vi "DI Remains.vi"(11 "DI":T1(array[cluster])) -> (2 "Same DI":T1(array[cluster]), 3 "Remains":T1(array[cluster]), 4 "DI Index":i32[](array[numeric]), 5 "DI value":bool[](array[boolean]))   [LabVIEW 2022 SP3]
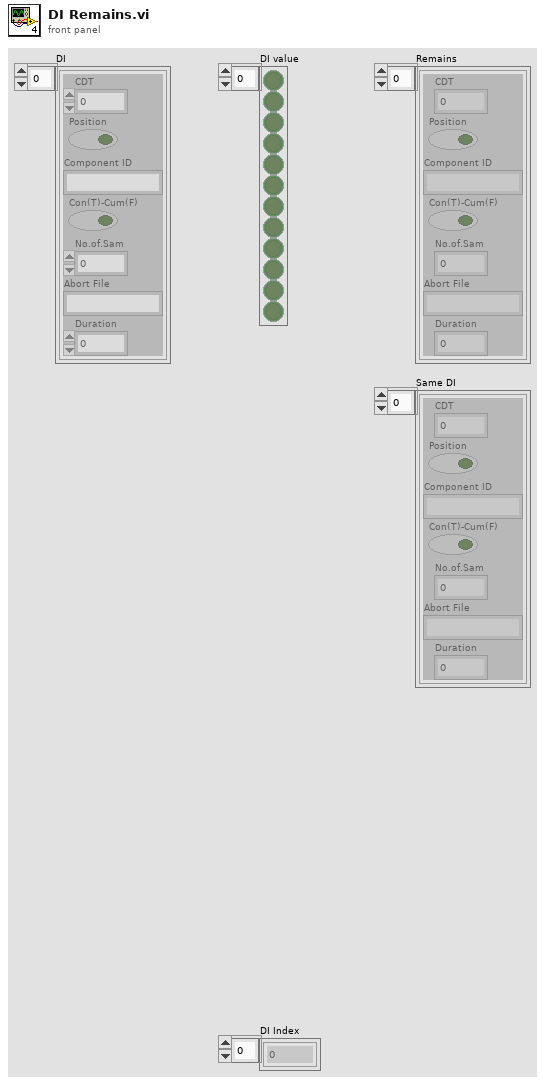
[diagram p1: front panel]
types:
  T1 = cluster{"CDT":dbl, "Position":bool, "Component ID":string, "Con(T)-Cum(F)":bool, "No.of.Sam":dbl, "Abort File":string, "Duration":u32}[]
  T2 = cluster{"CDT":dbl, "Position":bool, "Component ID":string, "Con(T)-Cum(F)":bool, "No.of.Sam":dbl, "Abort File":string, "Duration":u32}
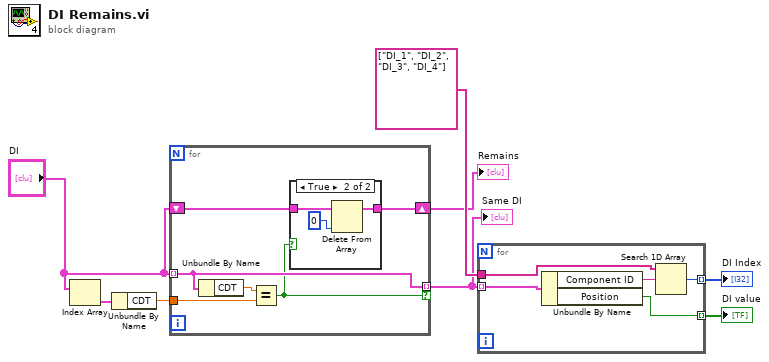
[diagram p0: block diagram]
diagram:
  n1 = Index Array(array="DI") -> (element=w2:T2)  [unwired: 1 in]
  n2 = Unbundle By Name(w2) -> ("CDT"=w1:dbl)
  n3 = for {
    tunnel: "DI" -> [w10] mode=indexing
    shift-right: [w13] -> w5
    shift-left: "DI" -> [w14]
    tunnel: w1 -> [w11]
    tunnel: [w10] -> w3 mode=indexing if=w9
    n4 = Unbundle By Name(w10) -> ("CDT"=w12:dbl)
    n5 = Equal?(x=w12, y=w11) -> (x = y?=w9:bool)
    n6 = case shown="True" w9 {
      tunnel: w14 -> [w15 w18]
      tunnel: [w15 w17] -> w13
      frame False {
      }
      frame True {
        n7 = Delete From Array(array=w18, index=0) -> (array with subset deleted=w17:T1)  [unwired: 1 in, 1 out]
      }
    }
  }
  "Remains" <- w5
  "Same DI" <- w3
  n8 = for {
    tunnel: w3 -> [w23] mode=indexing
    tunnel: string[] ["DI_1", "DI_2", "DI_3", "DI_4"] ("DO Names Out") -> [w22]
    tunnel: [w20] -> w7 mode=indexing
    tunnel: [w19] -> w8 mode=indexing
    n9 = Unbundle By Name(w23) -> ("Component ID"=w21:string, "Position"=w20:bool)
    n10 = Search 1D Array(1D array=w22, element=w21) -> (index of element=w19:i32)  [unwired: 1 in]
  }
  "DI value" <- w7
  "DI Index" <- w8
